vi "mhk_Trap-Incremental_corrected_dA2.vi"() -> ()   [LabVIEW 2010]
uses:
  <vilib>/Analysis/2dsp.llb/Integral Method.ctl
  <vilib>/Analysis/8numeric.llb/1D Numeric Integration.vi
  <vilib>/Analysis/NI_AALPro.lvlib
panel:
  out "delta x":dbl=0.5
  in  "derivative method":u16(ring)=2 items=["2nd Order Central", "4th Order Central", "Forward", "Backward"]
  out "dX/dt":dbl[](array[numeric])=[-0.5475824447462729, -2.1420349857947287, 21.63314273516883, -24.672601291251752, -0.02751321193894931]
  out "function vector":dbl[](array[numeric])=[2.8782945992814364, 2.6045033769083, 1.5334858840109356, 12.35005725159535, 0.013756605969474655]
  out "accumulated da vector":dbl[](array[numeric])=[0.0, 1.3706994940474342, 2.405196809277243, 5.876082593178815, 8.96703605757002]
  out "Integral X":dbl[](array[numeric])=[0.0, 1.3706994940474342, 2.405196809277243, 5.876082593178815, 8.967036057570022]
  out "raw da vector":dbl[](array[numeric])=[0.0, 1.3706994940474342, 1.034497315229809, 3.4708857839015717, 3.090953464391206]
  out "function\nvector\nsize":i32=5
  out "da\nvector\nsize":i32=5
  out "1D integration\nresult":dbl=8.96703605757002 format="%0.5f"
  out "Running Integral Graph":cluster{"Lower limit \"a\"":dbl, dbl, dbl[][]}(graph)={"Lower limit \"a\""=2.8, 0.5, [[0.0, 1.3706994940474342, 1.034497315229809, 3.4708857839015717, 3.090953464391206], [0.0, 1.3706994940474342, 2.405196809277243, 5.876082593178815, 8.96703605757002], [0.0, 1.3706994940474342, 2.405196809277243, 5.876082593178815, 8.967036057570022]]}
  in  "Plot BG Color":bool
  out "Approx. Integral \nover entire range\ndone incrementally":dbl=8.96703605757002
  out "Approx. Integral \nover entire range\ndone en masse":dbl=8.967036057570022
  out "Function Graph":cluster{"Lower limit \"a\"":dbl, dbl, dbl[]}(graph)={"Lower limit \"a\""=2.8, 0.5, [2.8782945992814364, 2.6045033769083, 1.5334858840109356, 12.35005725159535, 0.013756605969474655]}
  in  "Divisions \"N\"":dbl=4.0
  in  "Upper limit \"b\"":dbl=4.8
  in  "Lower limit \"a\"":dbl=2.8
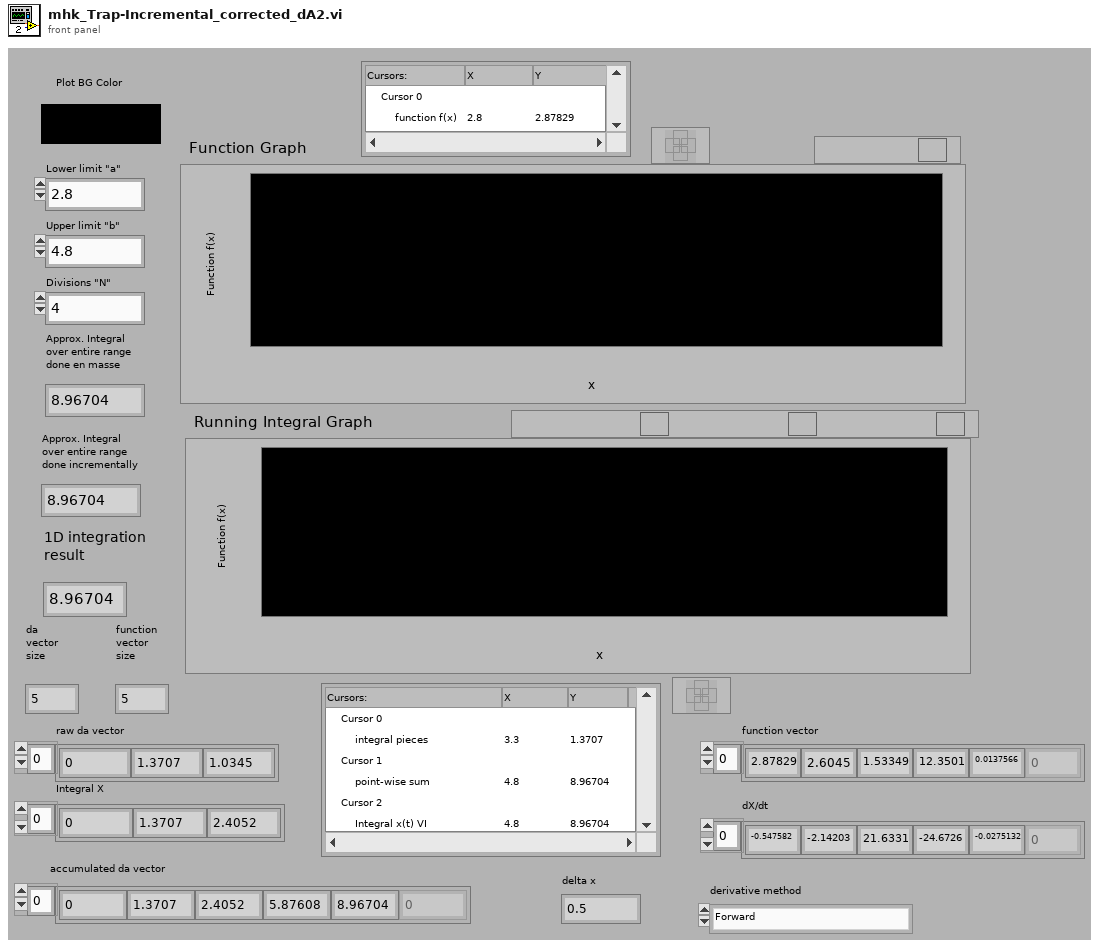
[diagram p1: front panel]
types:
  T1 = typedef "NI_AALPro.lvlib/Integral Method.ctl" = i32
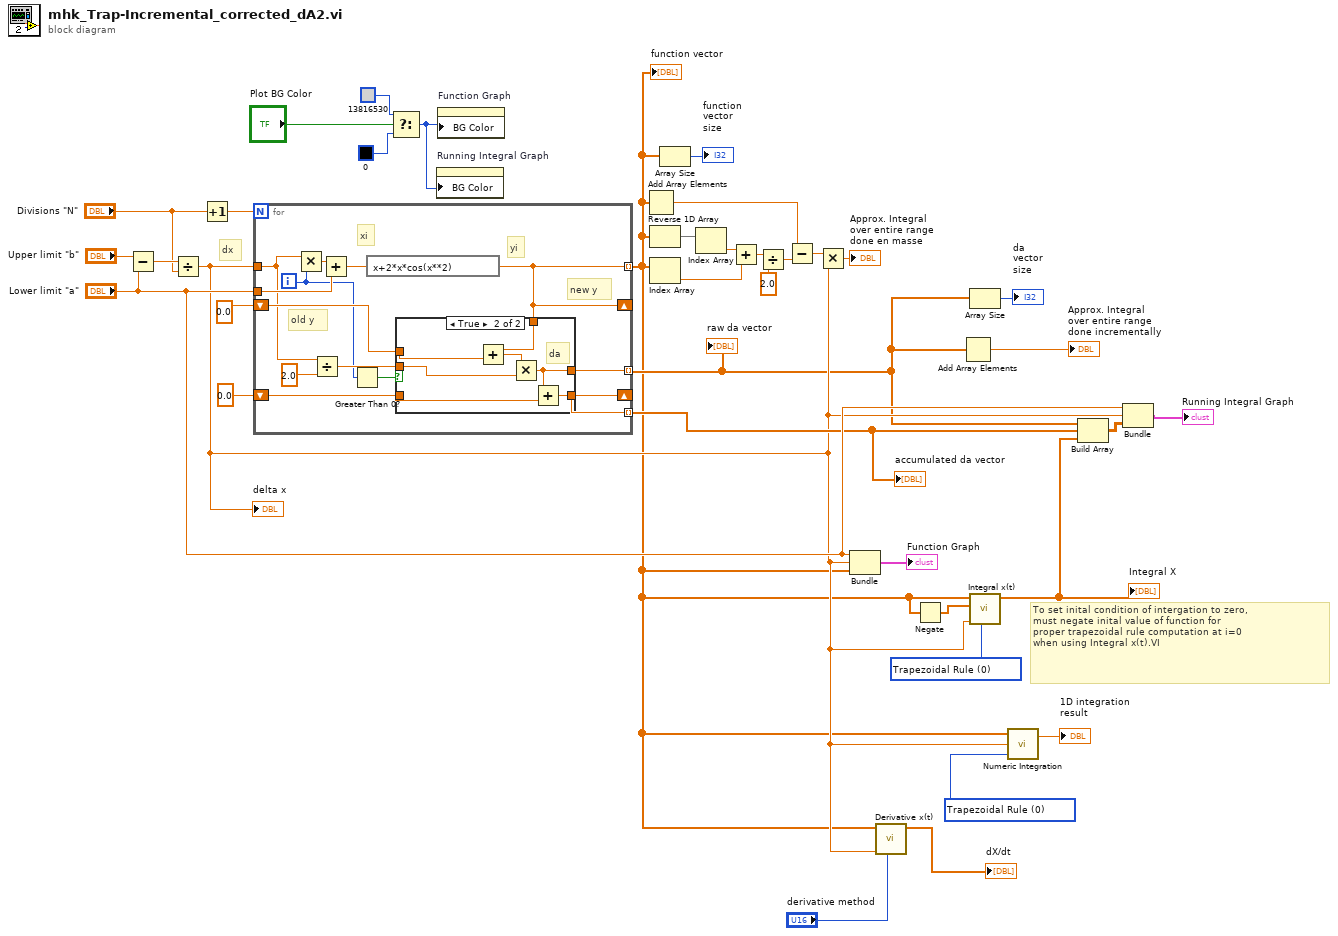
[diagram p0: block diagram]
diagram:
  w13 = T1 0 items=["Trapezoidal Rule", "Simpson's Rule", "Simpson's 3/8 Rule", "Bode Rule"] ("integration method")
  w15 = T1 0 items=["Trapezoidal Rule", "Simpson's Rule", "Simpson's 3/8 Rule", "Bode Rule"] ("integration method")
  # "To set inital condition of intergation to zero,\nmust negate inital value of function for \nproper trapezoidal rule computation at i=0 \nwhen using Integral x(t).VI"
  # "dx"
  n1 = Subtract(x="Upper limit \"b\"", y="Lower limit \"a\"") -> (x-y=w36:dbl)
  n2 = Divide(x=w36, y="Divisions \"N\"") -> (x/y=w12:dbl)
  "delta x" <- w12
  n3 = Increment(x="Divisions \"N\"") -> (x+1=w35:dbl)
  n4 = for {
    N: w35 -> [_]
    tunnel: w12 -> [w39]
    tunnel: "Lower limit \"a\"" -> [w49]
    tunnel: [w47] -> w4 mode=indexing
    shift-right: [w47] -> _
    shift-left: 0.0 -> [w46]
    tunnel: [w43] -> w5 mode=indexing
    shift-right: [w41] -> _
    shift-left: 0.0 -> [w42]
    tunnel: [w41] -> w17 mode=indexing
    i -> [w38]
    # "new y"
    # "old y"
    # "yi"
    # "xi"
    n5 = Multiply(x=w39, y=w38) -> (x*y=w50:dbl)
    n6 = Divide(x=w39, y=2.0) -> (x/y=w44:dbl)
    n7 = Add(x=w50, y=w49) -> (x+y=w48:dbl)
    n8 = Greater Than 0?(x=w38) -> (x > 0?=w40:bool)
    n9 = expression code="x+2*x*cos(x**2)"(w48) -> (w47:dbl)
    n10 = case shown="True" w40 {
      tunnel: w47 -> [_ w58]
      tunnel: w46 -> [_ w57]
      tunnel: w44 -> [_ w55]
      tunnel: [w51 w54] -> w43
      tunnel: w42 -> [w51 w53]
      tunnel: [w51 w52] -> w41
      frame False {
      }
      frame True {
        # "da"
        n11 = Add(x=w58, y=w57) -> (x+y=w56:dbl)
        n12 = Multiply(x=w56, y=w55) -> (x*y=w54:dbl)
        n13 = Add(x=w54, y=w53) -> (x+y=w52:dbl)
      }
    }
  }
  "raw da vector" <- w5
  "accumulated da vector" <- w17
  "function vector" <- w4
  n14 = Select(t=u32 13816530, s="Plot BG Color", f=u32 0) -> (s? t:f=w18:u32)
  n15 = property on="Running Integral Graph" class="WFGraph (strict)"("BG Color"=w18) -> ()  [unwired: 2 in, 2 out]
  n16 = property on="Function Graph" class="WFGraph (strict)"("BG Color"=w18) -> ()  [unwired: 2 in, 2 out]
  n17 = Add Array Elements(numeric array=w4) -> (sum=w27:dbl)
  n18 = Reverse 1D Array(array=w4) -> (reversed array=w33:dbl[])
  n19 = Index Array(array=w4) -> (element=w31:dbl)  [unwired: 1 in]
  n20 = Array Size(array=w4) -> (size(s)=→"function\nvector\nsize":i32)
  n21 = Index Array(array=w33) -> (element=w32:dbl)  [unwired: 1 in]
  n22 = Add(x=w32, y=w31) -> (x+y=w30:dbl)
  n23 = Divide(x=w30, y=2.0) -> (x/y=w28:dbl)
  n24 = Subtract(x=w27, y=w28) -> (x-y=w26:dbl)
  n25 = Multiply(x=w26, y=w12) -> (x*y=→"Approx. Integral \nover entire range\ndone en masse":dbl)
  n26 = Bundle("Lower limit \"a\""="Lower limit \"a\"", w12, w4) -> (→"Function Graph":cluster{"Lower limit \"a\"":dbl, dbl, dbl[]})  [unwired: 1 in]
  n27 = call <vilib>:"Derivative x(t).vi"("method"="derivative method", "dt"=w12, "X"=w4) -> ("dX/dt"=→"dX/dt":dbl[])  [unwired: 7 in, 1 out]
  n28 = Negate(x=w4) -> (-x=w3:dbl[])
  n29 = Add Array Elements(numeric array=w5) -> (sum=→"Approx. Integral \nover entire range\ndone incrementally":dbl)
  n30 = Array Size(array=w5) -> (size(s)=→"da\nvector\nsize":i32)
  n31 = call <vilib>:"Integral x(t).vi"("integration method"=w13, "dt"=w12, "Initial Condition"=w3, "X"=w4) -> ("Integral X"=w7:dbl[])  [unwired: 6 in, 1 out]
  "Integral X" <- w7
  n32 = call-poly <vilib>:"Numeric Integration.vi"("integration method"=w15, "dt"=w12, "Input Array"=w4) -> ("result"=→"1D integration\nresult":dbl)  [unwired: 1 out]
  n33 = Build Array(w5, w17, w7) -> (w16:dbl[][])
  n34 = Bundle("Lower limit \"a\""="Lower limit \"a\"", w12, w16) -> (→"Running Integral Graph":cluster{"Lower limit \"a\"":dbl, dbl, dbl[][]})  [unwired: 1 in]
